vi "Start Open Loop Scan.vi"(8 "error in (no error)":errorcluster, 10 "Scan Settings":T1, 11 "Context in":refnum<class "Context.lvclass">) -> (0 "error out":errorcluster, 3 "Context out":refnum<class "Context.lvclass">)   [LabVIEW 2015]
uses:
  Model/Model/Model.lvclass
  States/State/State.lvclass
  Context.lvclass
  Typedefs/Scan Settings.ctl
  Typedefs/FAMT Typedefs.lvlib
  Typedefs/Waveform Types.ctl
  Typedefs/Waveform Settings.ctl
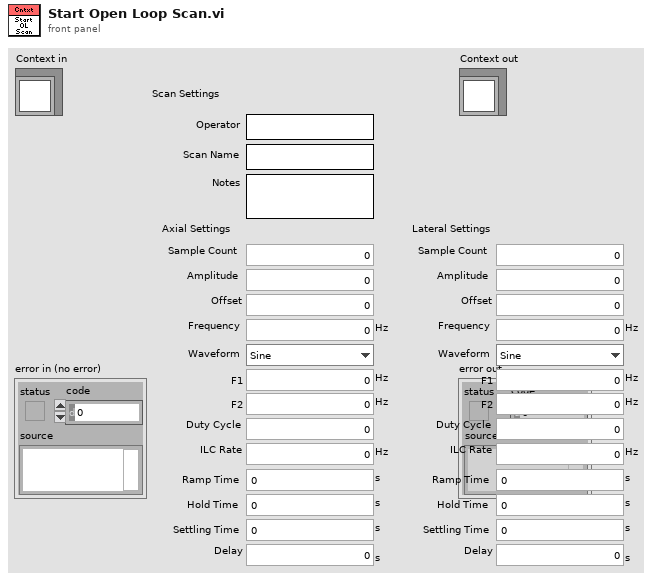
[diagram p1: front panel]
types:
  T1 = typedef "FAMT Typedefs.lvlib/Scan Settings.ctl" = cluster{"Operator":string, "Scan Name":string, "Notes":string, "Axial Settings":T2, "Lateral Settings":T2}
  T2 = typedef "FAMT Typedefs.lvlib/Waveform Settings.ctl" = cluster{"Sample Count":u32, "Amplitude":dbl, "Offset":dbl, "Frequency":dbl[unit], "Waveform":T3, "F1":dbl[unit], "F2":dbl[unit], "Duty Cycle":dbl, "ILC Rate":dbl[unit], "Ramp Time":dbl[unit], "Hold Time":dbl[unit], "Settling Time":dbl[unit], "Delay":dbl[unit]}
  T3 = typedef "FAMT Typedefs.lvlib/Waveform Types.ctl" = enum16{"Sine", "Triangle", "Square", "Sawtooth", "Chirp", "Gaussian", "Trapezoid"}
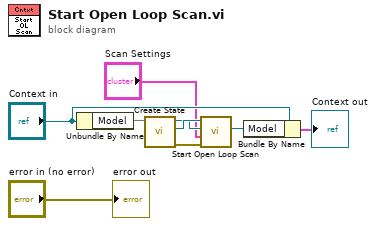
[diagram p0: block diagram]
diagram:
  n1 = Unbundle By Name("Context in") -> ("Model"=w8)
  n2 = call "Create State.vi"("Model in"=w8) -> ("error out"=w2:errorcluster, "State"=w4:refnum<class "State.lvclass">, "Model out"=w3:refnum<class "Model.lvclass">)  [unwired: 8 in]
  n3 = call-dynamic "Start Open Loop Scan.vi"("error in (no error)"=w2, "Scan Settings"="Scan Settings", "Model in"=w3, "State in"=w4) -> ("Model out"=w5:refnum<class "Model.lvclass">)  [unwired: 5 in, 2 out]
  n4 = Bundle By Name(cluster="Context in", "Model"=w5) -> (→"Context out":cluster{})
  "error out" <- "error in (no error)"
